vi "SuperVI2_0.vi"() -> ()   [LabVIEW 2021]
uses:
  <vilib>/MakerHub/LINX/Public/Peripherals/Digital/Digital Write 1 Chan.vi
  <vilib>/MakerHub/LINX/Public/Peripherals/Digital/Digital Write N Chans.vi
  <vilib>/MakerHub/LINX/Private/Local IO/LinxDigitalWrite.vi
  <vilib>/MakerHub/LINX/Public/Utilities/Check Channel.vi
  <vilib>/MakerHub/LINX/Public/Utilities/Open Serial.vi
  <vilib>/MakerHub/LINX/Private/Utilties/Generate Error.vi
  <vilib>/MakerHub/LINX/LMH-LINX.lvlib
panel:
  in  "STOP":bool
  in  "?":bool
  in  "?":bool
  in  "?":bool
  out "Absorption (%)":dbl[](graph)
  out "Transmission (%)":dbl[](graph)
  out "FILTER":dbl[](graph)
  in  "M1":bool
  in  "M0":bool
  in  "Motor steps":i32
  out "error out":errorcluster
  in  "Serial Port":refnum<visa-resource-name>="N/A"
  in  "error in (no error)":errorcluster
  out "LED":dbl[](graph)
  # "Function & M0 & M1\n ----------------------\nFull  Step:       0         0\n1/2   Step:       1         0\n1/8   Step:       0         1\n1/16 Step:       1         1"
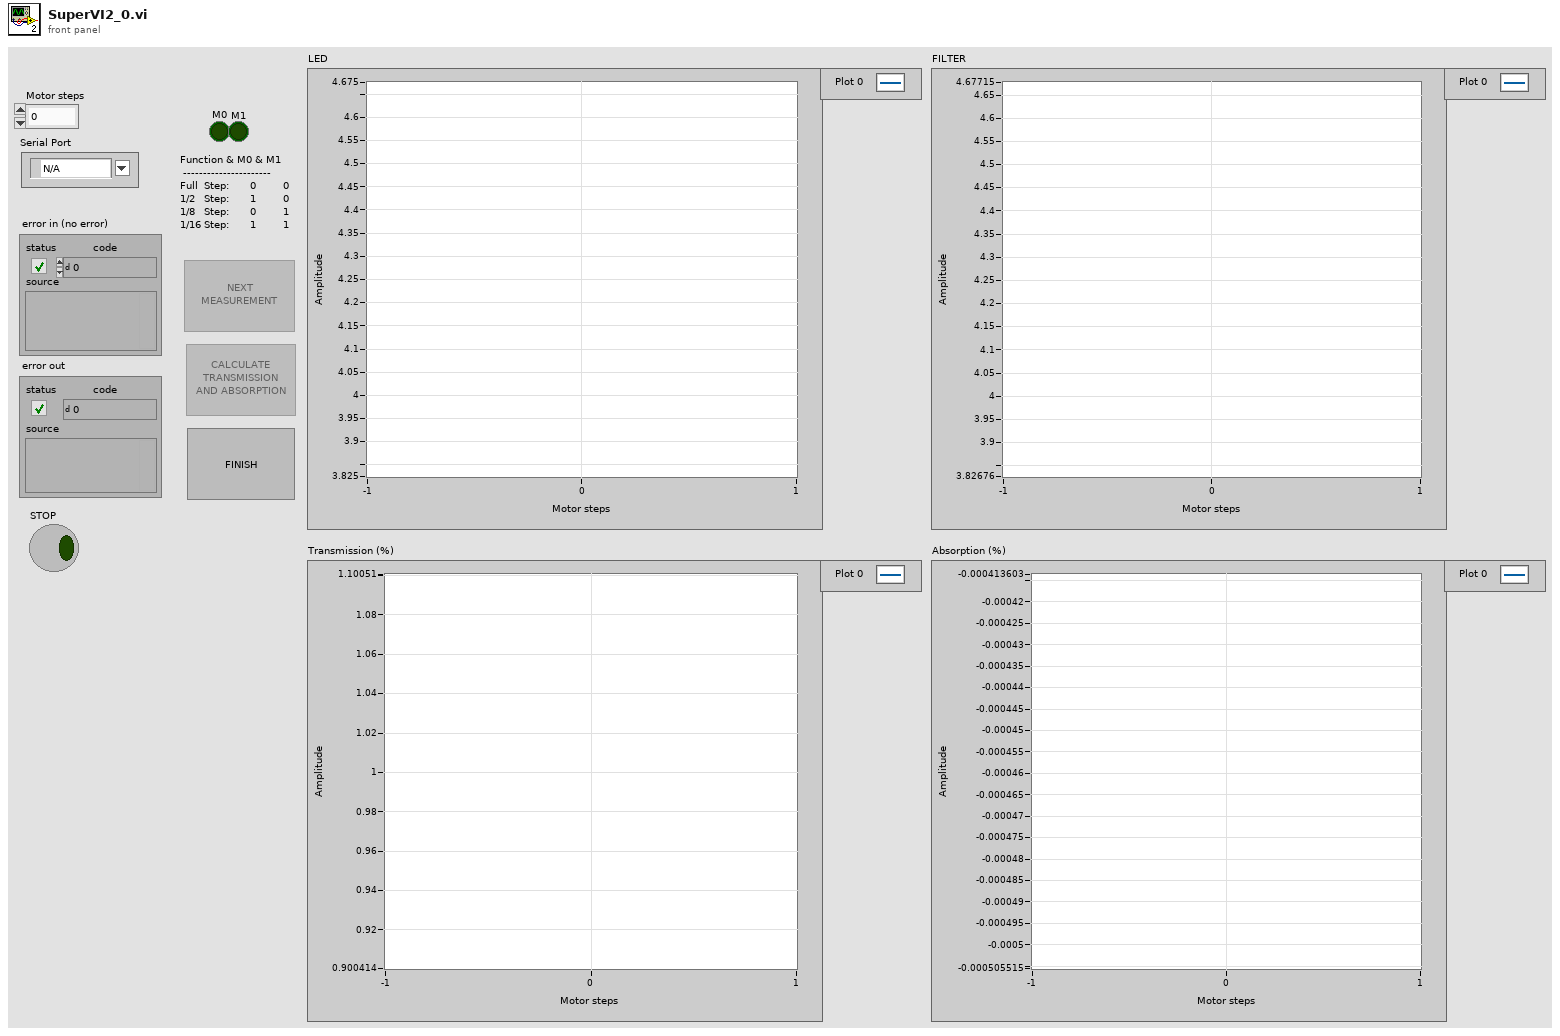
[diagram p1: front panel]
types:
  T1 = typedef "LMH-LINX.lvlib/LINX Ref.ctl" = cluster{"IO":T2, "Interface":T3, "LINX Device Config":T4}
  T2 = typedef "LMH-LINX.lvlib/Platform.ctl" = enum16{"Remote", "Local"}
  T3 = typedef "LMH-LINX.lvlib/Interface.ctl" = enum16{"Serial", "TCP"}
  T4 = typedef "LMH-LINX.lvlib/Device.lvlib/LINX Device Config.ctl" = cluster{"Interface":T3, "COM Port":refnum<visa-resource-name>, "TCP Configuration":T5, "Device Family":u8, "Device ID":u8, "Device Name":string, "TCP Ref":refnum<k5>, "Channels":T6}
  T5 = typedef "LMH-LINX.lvlib/Device.lvlib/TCP Config.ctl" = cluster{"IP Address":string, "Port":u16}
  T6 = typedef "LMH-LINX.lvlib/Channels.ctl" = cluster{"DI":u8[], "DO":u8[], "AI":u8[], "AO":u8[], "PWM":u8[], "QE":u8[], "UART":u8[], "I2C 2":u8[], "SPI":u8[], "CAN":u8[], "Servo":u8[], "AI Ref (V)":dbl, "AI Resolution (Bits)":u8, "AO Ref (V)":dbl, "AO Resolution (Bits)":u8}
  T7 = enum8{"Enabled", "Disabled", "Disabled and Grayed Out"}
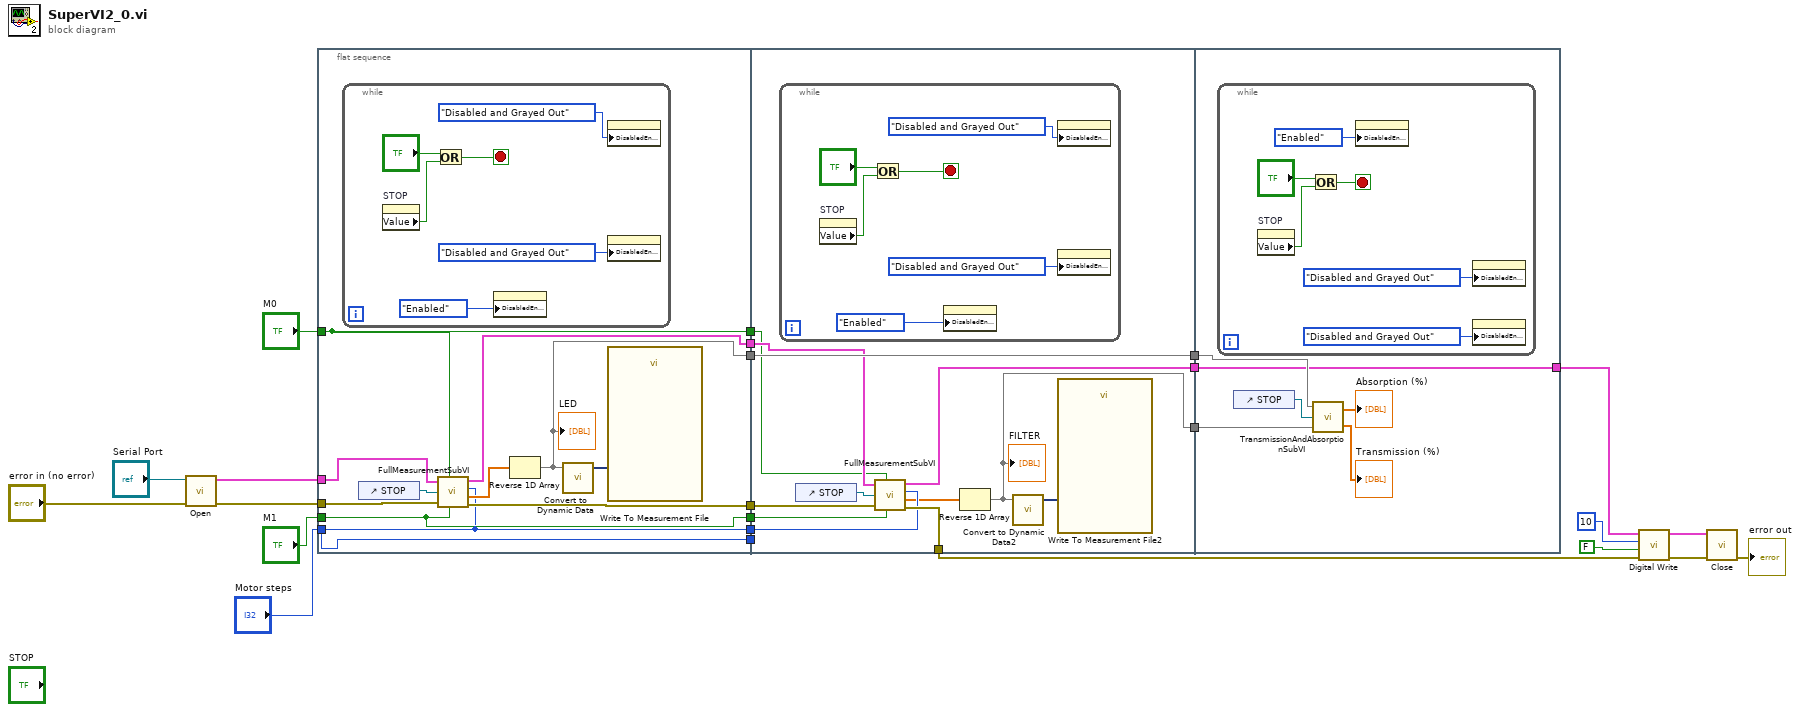
[diagram p0: block diagram]
diagram:
  n1 = call-poly <vilib>:"Open.vi"("Error In"="error in (no error)", "Serial Port"="Serial Port") -> ("Error Out"=w16:errorcluster, "LINX Resource"=w17:T1)  [unwired: 7 in, 1 out]
  n2 = flat-sequence {
    tunnel: w17 -> [w33]
    tunnel: w16 -> [w26]
    tunnel: "M0" -> [w29]
    tunnel: "M1" -> [w28]
    tunnel: "Motor steps" -> [w25]
    tunnel: [w29] -> w12
    tunnel: [w28] -> w11
    tunnel: [w25] -> w10
    tunnel: [w35] -> w8
    tunnel: [w32] -> w6
    tunnel: [w30] -> w5
    tunnel: [w25] -> w1
    tunnel: w12 -> [w44]
    tunnel: w11 -> [w45]
    tunnel: w10 -> [_]
    tunnel: [w53] -> w9
    tunnel: w8 -> [w53]
    tunnel: [w52] -> w7
    tunnel: w6 -> [w50]
    tunnel: w5 -> [w49]
    tunnel: [w48] -> w4
    tunnel: [w47] -> w2
    tunnel: w1 -> [w46]
    tunnel: w9 -> [w64]
    tunnel: w7 -> [w63]
    tunnel: [w60] -> w3
    tunnel: w2 -> [w60]
    frame #0 {
      n3 = while {
        stop <- w38 stop-if-true
        n4 = property on="STOP" class="Bool (strict)"() -> ("Value"=w36:bool)  [unwired: 2 in, 2 out]
        n5 = Or(x="?", y=w36) -> (x .or. y?=w38:bool)
        n6 = property class="Bool"("DisabledEnum"=T7."Enabled" ("Disabled")) -> ()  [unwired: 2 in, 2 out]
        n7 = property class="Bool"("DisabledEnum"=T7."Disabled and Grayed Out" ("Disabled")) -> ()  [unwired: 2 in, 2 out]
        n8 = property class="Bool"("DisabledEnum"=T7."Disabled and Grayed Out" ("Disabled")) -> ()  [unwired: 2 in, 2 out]
      }
      n9 = control-ref of="STOP"() -> (w27:refnum<vi>)
      n10 = call "FullMeasurementSubVI.vi"("LINX Resource"=w33, "M0"=w29, "Stop REF"=w27, "error in (no error)"=w26, "M1"=w28, "Motor steps"=w25) -> ("LINX Resource 2"=w32:T1, "Array"=w31:dbl[], "error out"=w30:errorcluster)
      n11 = Reverse 1D Array(array=w31) -> (reversed array=w35:dbl[])
      "LED" <- w35
      n12 = call "Convert to Dynamic Data"("Array"=w35) -> ("Dynamic Data Type"=w34:dynamicdata)  [unwired: 3 in]
      n13 = call "Write To Measurement File"("Signals"=w34) -> ()  [unwired: 16 in, 3 out]
    }
    frame #1 {
      n14 = while {
        stop <- w55 stop-if-true
        n15 = property on="STOP" class="Bool (strict)"() -> ("Value"=w56:bool)  [unwired: 2 in, 2 out]
        n16 = Or(x="?", y=w56) -> (x .or. y?=w55:bool)
        n17 = property class="Bool"("DisabledEnum"=T7."Enabled" ("Disabled")) -> ()  [unwired: 2 in, 2 out]
        n18 = property class="Bool"("DisabledEnum"=T7."Disabled and Grayed Out" ("Disabled")) -> ()  [unwired: 2 in, 2 out]
        n19 = property class="Bool"("DisabledEnum"=T7."Disabled and Grayed Out" ("Disabled")) -> ()  [unwired: 2 in, 2 out]
      }
      n20 = control-ref of="STOP"() -> (w42:refnum<vi>)
      n21 = call "FullMeasurementSubVI.vi"("LINX Resource"=w50, "M0"=w44, "Stop REF"=w42, "error in (no error)"=w49, "M1"=w45, "Motor steps"=w46) -> ("LINX Resource 2"=w47:T1, "Array"=w43:dbl[], "error out"=w48:errorcluster)
      n22 = Reverse 1D Array(array=w43) -> (reversed array=w52:dbl[])
      "FILTER" <- w52
      n23 = call "Convert to Dynamic Data2"("Array"=w52) -> ("Dynamic Data Type"=w51:dynamicdata)  [unwired: 3 in]
      n24 = call "Write To Measurement File2"("Signals"=w51) -> ()  [unwired: 16 in, 3 out]
    }
    frame #2 {
      n25 = while {
        stop <- w67 stop-if-true
        n26 = property on="STOP" class="Bool (strict)"() -> ("Value"=w66:bool)  [unwired: 2 in, 2 out]
        n27 = Or(x="?", y=w66) -> (x .or. y?=w67:bool)
        n28 = property class="Bool"("DisabledEnum"=T7."Enabled" ("Disabled")) -> ()  [unwired: 2 in, 2 out]
        n29 = property class="Bool"("DisabledEnum"=T7."Disabled and Grayed Out" ("Disabled")) -> ()  [unwired: 2 in, 2 out]
        n30 = property class="Bool"("DisabledEnum"=T7."Disabled and Grayed Out" ("Disabled")) -> ()  [unwired: 2 in, 2 out]
      }
      n31 = control-ref of="STOP"() -> (w65:refnum<vi>)
      n32 = call "TransmissionAndAbsorptionSubVI.vi"("array 2"=w63, "Stop REF"=w65, "array"=w64) -> ("appended array 2"=→"Transmission (%)":dbl[], "appended array"=→"Absorption (%)":dbl[])
    }
  }
  n33 = call-poly <vilib>:"Digital Write.vi"("Error In"=w4, "Output Value"=FALSE, "DO Channel"=u8 10, "LINX Resource"=w3) -> ("Error Out"=w18:errorcluster, "LINX Resource"=w19:T1)  [unwired: 6 in]
  n34 = call <vilib>:"Close.vi"("Error In"=w18, "LINX Resource"=w19) -> ("Error Out"=→"error out":errorcluster)  [unwired: 9 in]
